vi "constructor.vi"() -> (0 "error out":errorcluster, 3 "new reference":refnum<k24>)   [LabVIEW 2024]
uses:
  D:/git/Sourcegrid-LabVIEW/dll/SourceGrid.dll
  SourceGrid.dll
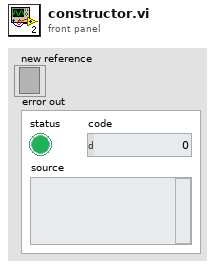
[diagram p1: front panel]
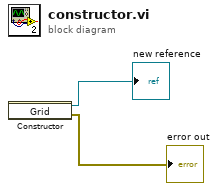
[diagram p0: block diagram]
diagram:
  n1 = constructor class="Grid"() -> (reference out=→"new reference":refnum<k24>, error out=→"error out":errorcluster)  [unwired: 3 in, 1 out]
